vi "题目5.vi"() -> ()   [LabVIEW 2017]
panel:
  out "显示面板":T1 {"油量" scale=0.0..200.0; "转速（r/s）" scale=0.0..8000.0; "速度（Km/h）" scale=0.0..300.0}
  in  "停止":bool
  out "油量报警":bool
  in  "控制面板":T2 {"档位" scale=0.0..10.0; "油门" scale=0.0..10.0}
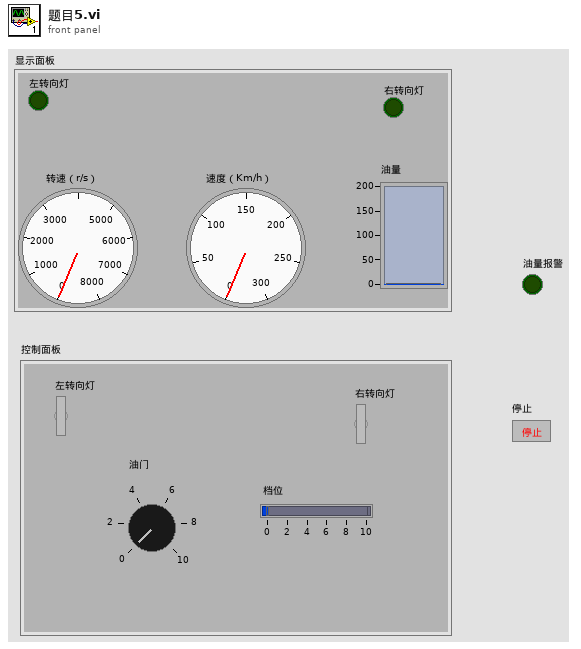
[diagram p1: front panel]
types:
  T1 = cluster{"左转向灯":bool, "右转向灯":bool, "转速（r/s）":dbl, "速度（Km/h）":dbl, "油量":dbl}
  T2 = cluster{"左转向灯":bool, "右转向灯":bool, "油门":dbl, "档位":dbl}
  T3 = cluster{"左转向灯":bool, "右转向灯":bool, dbl, dbl, "b":dbl}
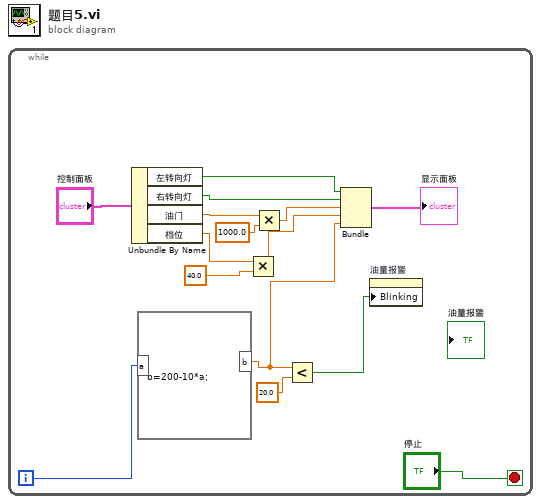
[diagram p0: block diagram]
diagram:
  n1 = while {
    i -> [w5]
    stop <- "停止" stop-if-true
    n2 = Unbundle By Name("控制面板") -> ("左转向灯"=w14:bool, "右转向灯"=w13:bool, "油门"=w12:dbl, "档位"=w9:dbl)
    n3 = formula code="b=200-10*a;"("a"=w5) -> ("b"=w3:dbl)
    n4 = Multiply(x=w9, y=40.0) -> (x*y=w7:dbl)
    n5 = Multiply(x=w12, y=1000.0) -> (x*y=w10:dbl)
    n6 = Less?(x=w3, y=20.0) -> (x < y?=w1:bool)
    n7 = Bundle("左转向灯"=w14, "右转向灯"=w13, w10, w7, "b"=w3) -> (→"显示面板":T3)  [unwired: 1 in]
    n8 = property on="油量报警" class="Bool (严格)"("Blinking"=w1) -> ()  [unwired: 2 in, 2 out]
  }
